vi "StringToI8[](cast).vi"(1 "String":string) -> (0 "I8[]":i8[](array[numeric]))   [LabVIEW 2012]
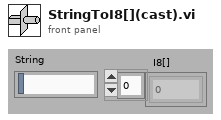
[diagram p1: front panel]
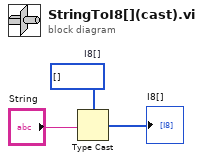
[diagram p0: block diagram]
diagram:
  w2 = i8[] []  # I8[]
  n1 = Type Cast(type=w2, x="String") -> (*(type *) &x=→"I8[]":i8[])
